vi "Intan_AmpInfo.vi"(3 "error in":errorcluster, 4 "byte count":u32=1000, 5 "VISA resource name":refnum<visa-resource-name>) -> (0 "error out":errorcluster, 1 "ampInfoTextResponse":string, 2 "VISA resource name out":refnum<visa-resource-name>)   [LabVIEW 2020]
doc: "This VI queries the Intan RHD2000 chip for revision history, die revision, and number amplifiers."
panel:
  out "return count spi1":u32
  out "response spi1":string
  out "return count spi0":u32
  out "response spi0":string
  in  "Teensy event char":string="i"
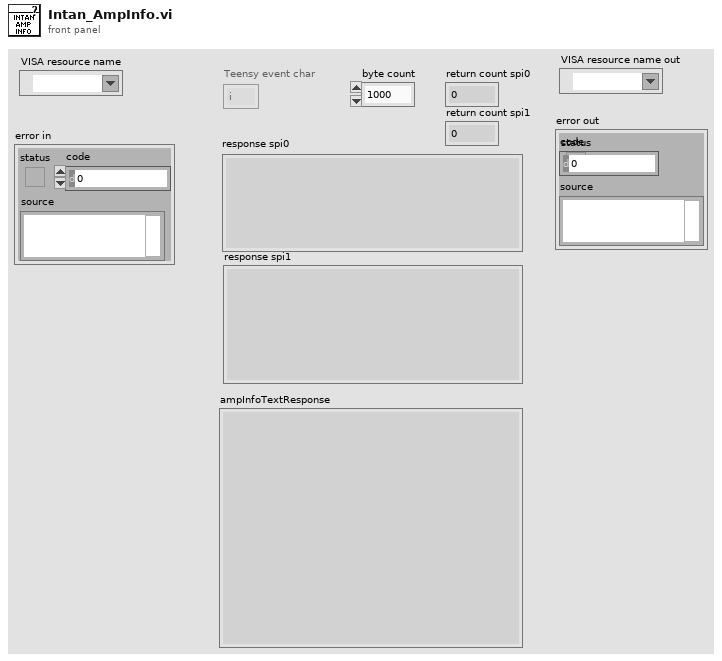
[diagram p1: front panel]
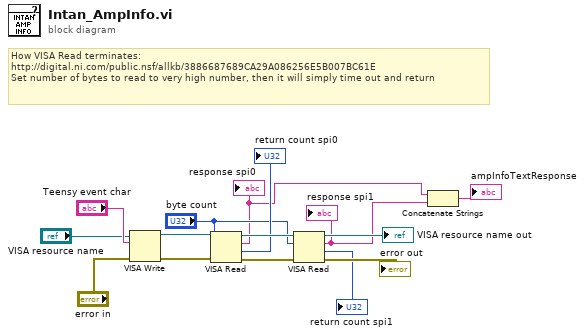
[diagram p0: block diagram]
diagram:
  # "How VISA Read terminates:\nhttp://digital.ni.com/public.nsf/allkb/3886687689CA29A086256E5B007BC61E\nSet number of bytes to read to very high number, then it will simply time out and return"
  n1 = VISA Write(VISA resource name="VISA resource name", write buffer="Teensy event char", error in (no error)="error in") -> (VISA resource name out=w10:refnum<visa-resource-name>, error out=w9:errorcluster)  [unwired: 1 out]
  n2 = VISA Read(VISA resource name=w10, byte count="byte count", error in (no error)=w9) -> (VISA resource name out=w14:refnum<visa-resource-name>, read buffer=w2:string, return count=→"return count spi0":u32, error out=→"error out":errorcluster)
  "response spi0" <- w2
  n3 = VISA Read(VISA resource name=w14, byte count="byte count") -> (VISA resource name out=→"VISA resource name out":refnum<visa-resource-name>, read buffer=w3:string, return count=→"return count spi1":u32)  [unwired: 1 in, 1 out]
  "response spi1" <- w3
  n4 = Concatenate Strings(w2, w3) -> (→"ampInfoTextResponse":string)
